vi "Check Angle in Range.vi"(2 "CW(-1)/CCW(1)":dbl, 3 "Angle to Next Destination":dbl, 4 "Angle Threshold":dbl=10.0) -> (0 "Left/Right":string, 1 "Angle in Range?":bool)   [LabVIEW 2011]
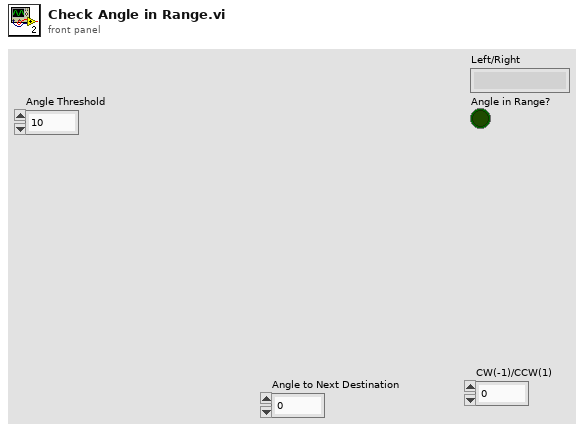
[diagram p1: front panel]
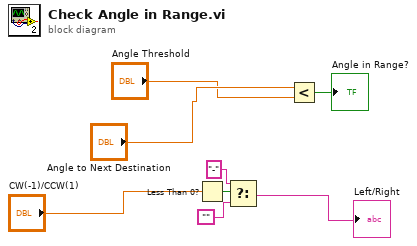
[diagram p0: block diagram]
diagram:
  n1 = Less Than 0?(x="CW(-1)/CCW(1)") -> (x < 0?=w7:bool)
  n2 = Select(t="-", s=w7, f="") -> (s? t:f=→"Left/Right":string)
  n3 = Less?(x="Angle to Next Destination", y="Angle Threshold") -> (x < y?=→"Angle in Range?":bool)
